vi "DigitalOutput.vi"(8 "error in (no error)":errorcluster, 11 "Queue in":refnum<queue>) -> (0 "error out":errorcluster)   [LabVIEW 2018]
uses:
  Controls/Enums/DigiLoopEnum.ctl
  Controls/Clusts/DigOutClust.ctl
  <vilib>/DAQmx/write.llb/DAQmx Write (Digital 1D Bool NChan 1Samp 1Line).vi
  <vilib>/DAQmx/create/channels.llb/DAQmx Create Channel (DO-Digital Output).vi
  <vilib>/DAQmx/miscellaneous.llb/DAQmx Fill In Error Info.vi
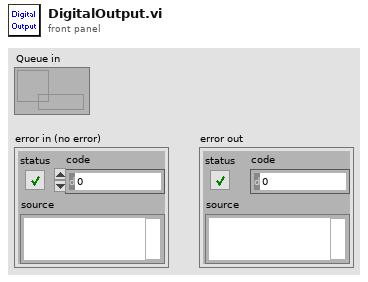
[diagram p1: front panel]
types:
  T1 = typedef "DigOutClust.ctl" = cluster{"Green":bool, "Rx_Yell":bool, "Cx_Yell":bool, "Red":bool, "Source":string}
  T2 = typedef "DigiLoopEnum.ctl" = enum16{"Dig_Init", "Digi_Write", "Digi_Exit"}
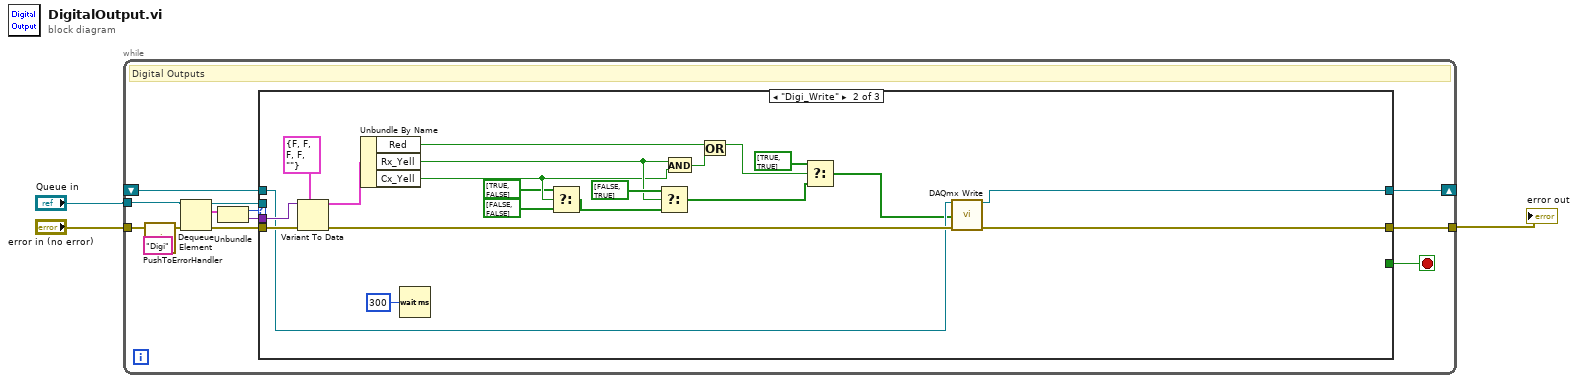
[diagram p0: block diagram]
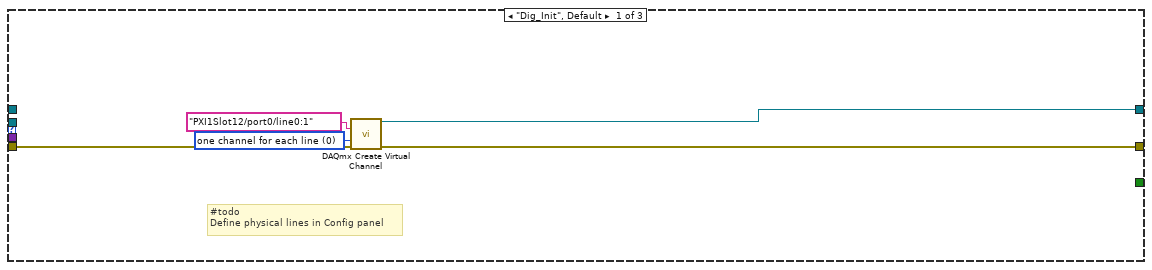
[diagram p2: hidden frame]
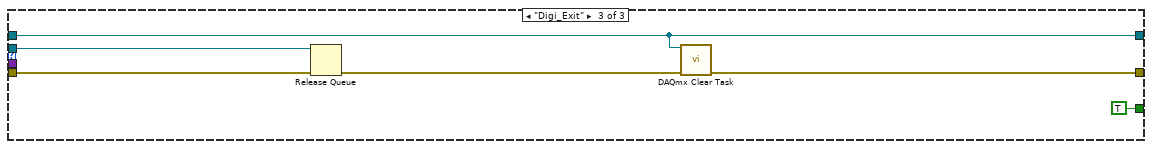
[diagram p3: hidden frame]
diagram:
  n1 = while {
    tunnel: "Queue in" -> [w7]
    tunnel: "error in (no error)" -> [w10]
    tunnel: [w16] -> w3
    shift-right: [w15] -> _
    shift-left: _ -> [w4]
    stop <- w14 stop-if-true
    # "Digital Outputs"
    n2 = call "PushToErrorHandler.vi"("ErrorIn"=w10, "ErrorLocation"="Digi") -> ("ErrorOut"=w12:errorcluster)  [unwired: 5 in]
    n3 = Dequeue Element(queue=w7, error in (no error)=w12) -> (queue out=w6:refnum<queue>, element=w11:cluster{"Enum":T2, "Data":variant}, error out=w9:errorcluster)  [unwired: 1 in, 1 out]
    n4 = Unbundle(w11) -> ("Enum"=w8:T2, "Data"=w5:variant)
    n5 = case shown="\"Digi_Write\"" w8 {
      tunnel: w9 -> [w17 w39 w47]
      tunnel: [w19 w42 w44] -> w16
      tunnel: [w18 w41 w43] -> w15
      tunnel: [_ _ TRUE ("Exit")] -> w14
      tunnel: w6 -> [_ _ w46]
      tunnel: w5 -> [_ w37 _]
      tunnel: w4 -> [_ w28 w43]
      frame "Dig_Init", Default {
        w20 = 0 items=["one channel for each line", "one channel for all lines"] ("line grouping")
        # "#todo\nDefine physical lines in Config panel"
        n6 = call-poly <vilib>:"DAQmx Create Virtual Channel.vi"("lines"=tag "PXI1Slot12/port0/line0:1", "line grouping"=w20, "error in"=w17) -> ("task out"=w18:refnum<k21>, "error out"=w19:errorcluster)  [unwired: 11 in]
      }
      frame "Digi_Write" {
        n7 = Variant To Data(error in=w39, type=T1 {"Green"=FALSE, "Rx_Yell"=FALSE, "Cx_Yell"=FALSE, "Red"=FALSE, "Source"=""} ("DigOut"), Variant=w37) -> (data=w35:T1, error out=w38:errorcluster)
        n8 = Unbundle By Name(w35) -> ("Red"=w33:bool, "Rx_Yell"=w27:bool, "Cx_Yell"=w26:bool)
        n9 = Wait (ms)(milliseconds to wait=u32 300) -> ()  [unwired: 1 out]
        n10 = Select(t=bool[] [TRUE, FALSE] ("data"), s=w26, f=bool[] [FALSE, FALSE] ("data")) -> (s? t:f=w22:bool[])
        n11 = Select(t=bool[] [FALSE, TRUE] ("data"), s=w27, f=w22) -> (s? t:f=w30:bool[])
        n12 = And(x=w27, y=w26) -> (x .and. y?=w31:bool)
        n13 = Or(x=w33, y=w31) -> (x .or. y?=w32:bool)
        n14 = Select(t=bool[] [TRUE, TRUE] ("data"), s=w32, f=w30) -> (s? t:f=w23:bool[])
        n15 = call-poly <vilib>:"DAQmx Write.vi"("task/channels in"=w28, "data"=w23, "error in"=w38) -> ("task out"=w41:refnum<k21>, "error out"=w42:errorcluster)  [unwired: 10 in, 1 out]
      }
      frame "Digi_Exit" {
        n16 = Release Queue(queue=w46, error in (no error)=w47) -> (error out=w45:errorcluster)  [unwired: 1 in, 2 out]
        n17 = call <vilib>:"DAQmx Clear Task.vi"("task in"=w43, "error in"=w45) -> ("error out"=w44:errorcluster)  [unwired: 13 in]
      }
    }
  }
  "error out" <- w3
